vi "REST_req.vi"(5 "Request":T2(ring), 6 "Multipart Data In":T1[](array[typedef])=[{"Name"="imageblock1", "Value"="Collectable", "File"=path "C:/Users/monke/Desktop/Work/VIs to modify/ONENOTE/Sandbox/curl-logo.png", "Filename"="curl-logo.png", "MIME type"="image/png"}, {"Name"="content", "Value"="swagmaster flash", "File"=path "", "Filename"="Nothing", "MIME type"="image/png"}], 7 "Headers In":cluster{"Name":string, "Value":string}[](array[cluster]), 8 "error in":errorcluster, 9 "Body":string, 10 "Content-Type":string, 11 "URL":string) -> (0 "error out":errorcluster, 2 "ERROR":string, 3 "OUTPUT":string)   [LabVIEW 2016]
uses:
  <vilib>/httpClient/MultipartData.ctl
  <vilib>/httpClient/LabVIEWHTTPClient.lvlib
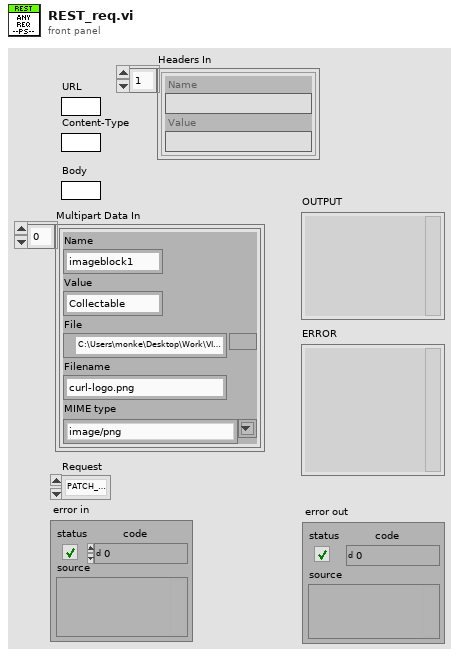
[diagram p1: front panel]
types:
  T1 = typedef "LabVIEWHTTPClient.lvlib/MultipartData.ctl" = cluster{"Name":string, "Value":string, "File":path, "Filename":string, "MIME type":string}
  T2 = enum16{"PATCH_MULTIPART", "POST_MULTIPART", "PATCH", "DELETE", "HEAD", "PUT", "GET"}
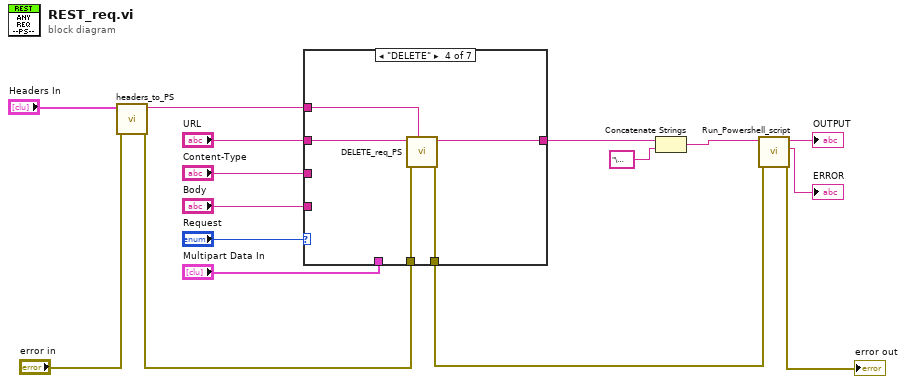
[diagram p0: block diagram]
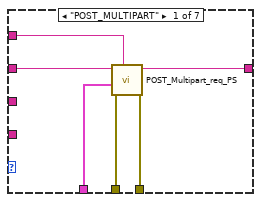
[diagram p2: hidden frame]
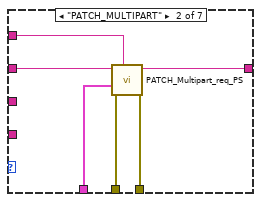
[diagram p3: hidden frame]
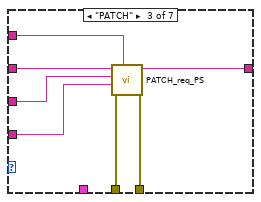
[diagram p4: hidden frame]
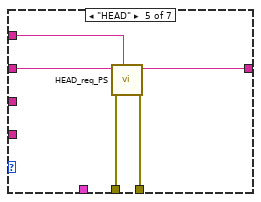
[diagram p5: hidden frame]
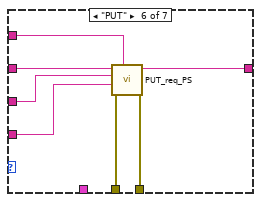
[diagram p6: hidden frame]
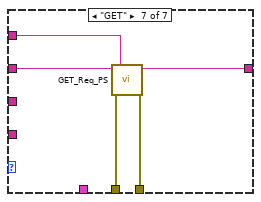
[diagram p7: hidden frame]
diagram:
  n1 = call "headers_to_PS.vi"("error in"="error in", "Headers In"="Headers In") -> ("error out"=w2:errorcluster, "Headers_PS_Dict"=w4:string)  [unwired: 8 in]
  n2 = case shown="\"DELETE\"" "Request" {
    tunnel: "Multipart Data In" -> [w22 w28 _ _ _ _ _]
    tunnel: "URL" -> [w19 w27 w35 w37 w43 w52 w54]
    tunnel: w2 -> [w21 w23 w34 w40 w45 w49 w55]
    tunnel: [w20 w24 w33 w39 w44 w48 w56] -> w11
    tunnel: w4 -> [w18 w26 w32 w36 w42 w47 w53]
    tunnel: [w17 w25 w29 w38 w41 w46 w57] -> w5
    tunnel: "Content-Type" -> [_ _ w30 _ _ w51 _]
    tunnel: "Body" -> [_ _ w31 _ _ w50 _]
    frame "POST_MULTIPART" {
      n3 = call "POST_Multipart_req_PS.vi"("Headers"=w18, "error in"=w21, "Multipart Data In"=w22, "URL"=w19) -> ("error out"=w20:errorcluster, "Multipart PATCH Request"=w17:string)  [unwired: 6 in]
    }
    frame "PATCH_MULTIPART" {
      n4 = call "PATCH_Multipart_req_PS.vi"("Headers"=w26, "error in"=w23, "Multipart Data In"=w28, "URL"=w27) -> ("error out"=w24:errorcluster, "Multipart PATCH Request"=w25:string)  [unwired: 6 in]
    }
    frame "PATCH" {
      n5 = call "PATCH_req_PS.vi"("Headers"=w32, "error in"=w34, "Body"=w31, "ContentType"=w30, "URL"=w35) -> ("error out"=w33:errorcluster, "PATCH Request"=w29:string)  [unwired: 5 in]
    }
    frame "DELETE" {
      n6 = call "DELETE_req_PS.vi"("Headers"=w36, "error in"=w40, "URL"=w37) -> ("error out"=w39:errorcluster, "DELETE Request"=w38:string)  [unwired: 7 in]
    }
    frame "HEAD" {
      n7 = call "HEAD_req_PS.vi"("Headers"=w42, "error in"=w45, "URL"=w43) -> ("error out"=w44:errorcluster, "HEAD Request"=w41:string)  [unwired: 7 in]
    }
    frame "PUT" {
      n8 = call "PUT_req_PS.vi"("Headers"=w47, "error in"=w49, "ContentType"=w50, "Body"=w51, "URL"=w52) -> ("error out"=w48:errorcluster, "PUT Request"=w46:string)  [unwired: 5 in]
    }
    frame "GET" {
      n9 = call "GET_Req_PS.vi"("Headers"=w53, "error in"=w55, "URL"=w54) -> ("error out"=w56:errorcluster, "GET Request"=w57:string)  [unwired: 7 in]
    }
  }
  n10 = Concatenate Strings(w5, "\nWrite-Host \"StatusCode\"\nWrite-Host \"START\"\n$request.StatusCode\nWrite-Host \"END\"\nWrite-Host \"StatusDescription\"\nWrite-Host \"START\"\n$request.StatusDescription\nWrite-Host \"END\"\nWrite-Host \"Headers\"\nWrite-Host \"START\"\n$request.headers | convertto-json\nWrite-Host \"END\"\nWrite-Host \"RawContent\"\nWrite-Host \"START\"\n$request.content\nWrite-Host \"END\"" ("string")) -> (w6:string)
  n11 = call "Run_Powershell_script.vi"("error in"=w11, "Powershell Script"=w6) -> ("error out"=→"error out":errorcluster, "standard error"=→"ERROR":string, "standard output"=→"OUTPUT":string)  [unwired: 7 in]
